vi "Broadcast Item Key.vi"(3 "Status":string="status", 4 "Target":string="target", 5 "Source":string="source") -> (2 "Key":string="status@source->target")   [LabVIEW 2017, in "Communicable State Machine.lvlib"]
doc: "### Broadcast Item Key.vi\n\n-- <b>Controls</b> --\n- <b>status</b>:\n- <b>target</b>:\n- <b>source</b>:\n\n-- <b>Indicators</b> --\n- <b>key</b>:"
uses:
  Communicable State Machine.lvlib
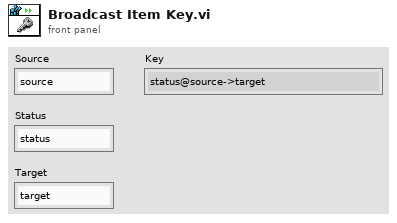
[diagram p1: front panel]
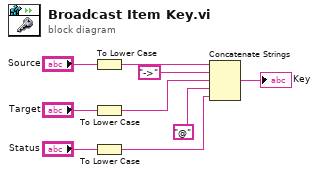
[diagram p0: block diagram]
diagram:
  n1 = To Lower Case(string="Source") -> (all lower case string=w8:string)
  n2 = To Lower Case(string="Target") -> (all lower case string=w3:string)
  n3 = To Lower Case(string="Status") -> (all lower case string=w1:string)
  n4 = Concatenate Strings(w8, "->" ("string"), w3, "@" ("string"), w1) -> (→"Key":string)
